vi "Mcp2210 Get Spi Status.vi"(8 "error in (no error)":errorcluster, 11 "handle":i32) -> (0 "error out":errorcluster, 2 "SPI Status":T1, 3 "handle out":i32)   [LabVIEW 2015, in "mcp2210.lvlib"]
doc: "If there is no device communication error, this command returns 0 (E_SUCCESS) and\nupdates the pointers with information about SPI transfer status. In case of error, the function\nreturns negative error code.\nParameters:\nInputs:\n- void *handle - The pointer to the USB device handle. Cannot be NULL.\nOutputs:\n- unsigned char *pspiExtReqStat - SPI Bus release external request status:\n- 0x01 ¨C No External Request for SPI Bus Release\n- 0x00 ¨C Pending External Request for SPI Bus Release\nCannot be NULL.\n- unsigned char *pspiOwner - SPI Bus current owner:\n- 0x00 - No owner\n- 0x01 - USB Bridge\n- 0x02 - External Master.\nCannot be NULL.\n- unsigned char *pspiTxferStat - SPI transfer status:\n- 0x00 - No SPI transfer in progress\n- 0x01 - SPI transfer is in progress\nCannot be NULL.\nReturns:\n- 0 for success: E_SUCCESS\n- negative error code: E_ERR_NULL, E_ERR_INVALID_HANDLE_VALUE\nE_ERR_HID_TIMEOUT, E_ERR_HID_RW_FILEIO, E_ERR_UNKOWN_ERROR\nE_ERR_CMD_ECHO, E_ERR_CMD_FAILED\n\nMCP2210_DLL_UM_API int __stdcall Mcp2210_GetSpiStatus(void *handle, unsigned char *pspiExtReqStat, unsigned char *pspiOwner, unsigned char *pspiTxferStat);"
uses:
  <userlib>/mcp2210/mcp2210.lvlib
  <userlib>/mcp2210/mcp2210_dll_um_x86.dll
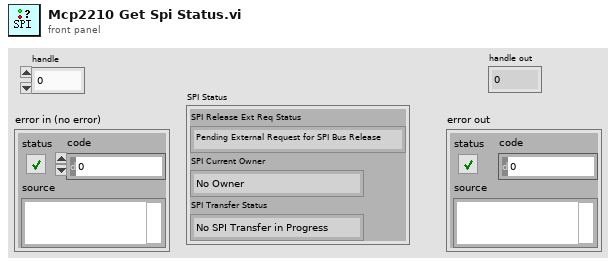
[diagram p1: front panel]
types:
  T1 = cluster{"SPI Release Ext Req Status":enum16{"Pending External Request for SPI Bus Release", "No External Request for SPI Bus Release"}, "SPI Current Owner":enum16{"No Owner", "USB Bridge", "External Master"}, "SPI Transfer Status":enum16{"No SPI Transfer in Progress", "SPI Transfer in Progress"}}
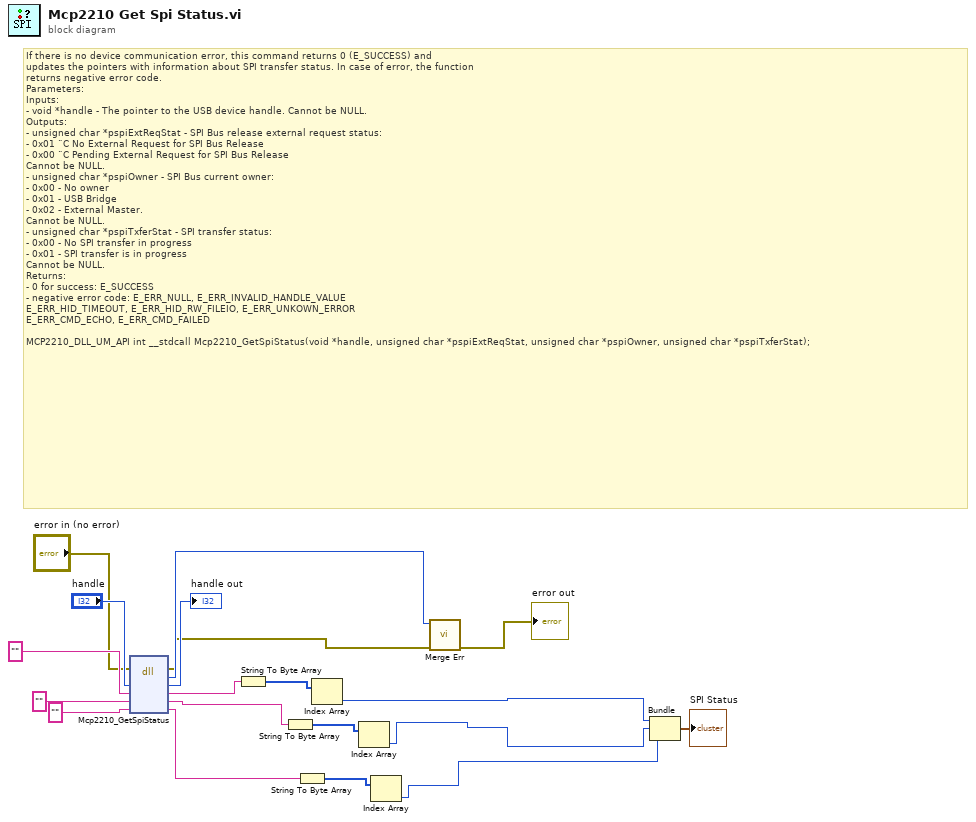
[diagram p0: block diagram]
diagram:
  # "If there is no device communication error, this command returns 0 (E_SUCCESS) and\nupdates the pointers with information about SPI transfer status. In case of error, the function\nreturns negative error code.\nParameters:\nInputs:\n- void *handle - The pointer to the USB device handle. Cannot be NULL.\nOutputs:\n- unsigned char *pspiExtReqStat - SPI Bus release external request status:\n- 0x01 ¨C No External Request for SPI Bus Release\n- 0x00 ¨C Pending External Request for SPI Bus Release\nCannot be NULL.\n- unsigned char *pspiOwner - SPI Bus current owner:\n- 0x00 - No owner\n- 0x01 - USB Bridge\n- 0x02 - External Master.\nCannot be NULL.\n- unsigned char *pspiTxferStat - SPI transfer status:\n- 0x00 - No SPI transfer in progress\n- 0x01 - SPI transfer is in progress\nCannot be NULL.\nReturns:\n- 0 for success: E_SUCCESS\n- negative error code: E_ERR_NULL, E_ERR_INVALID_HANDLE_VALUE\nE_ERR_HID_TIMEOUT, E_ERR_HID_RW_FILEIO, E_ERR_UNKOWN_ERROR\nE_ERR_CMD_ECHO, E_ERR_CMD_FAILED\n\nMCP2210_DLL_UM_API int __stdcall Mcp2210_GetSpiStatus(void *handle, unsigned char *pspiExtReqStat, unsigned char *pspiOwner, unsigned char *pspiTxferStat);"
  n1 = dll-call lib="D:/LabVIEW 2015/user.lib/mcp2210/mcp2210_dll_um_x86.*" fn="Mcp2210_GetSpiStatus"(error in="error in (no error)", "handle"="handle", "pspiExtReqStat"="", "pspiOwner"="", "pspiTxferStat"="") -> (error out=w13:errorcluster, "return type"=w14:i32, "handle"=→"handle out":i32, "pspiExtReqStat"=w10:string, "pspiOwner"=w7:string, "pspiTxferStat"=w5:string)  [unwired: 2 in, 1 out]
  n2 = String To Byte Array(string=w10) -> (unsigned byte array=w9:u8[])
  n3 = String To Byte Array(string=w7) -> (unsigned byte array=w8:u8[])
  n4 = String To Byte Array(string=w5) -> (unsigned byte array=w6:u8[])
  n5 = Index Array(array=w9) -> (element=w4:u8)  [unwired: 1 in]
  n6 = Index Array(array=w8) -> (element=w3:u8)  [unwired: 1 in]
  n7 = Index Array(array=w6) -> (element=w2:u8)  [unwired: 1 in]
  n8 = call <userlib>:"Merge Err.vi"("error in (no error)"=w13, "return type"=w14) -> ("error out"=→"error out":errorcluster)  [unwired: 9 in]
  n9 = Bundle(w4, w3, w2) -> (→"SPI Status":cluster{u8, u8, u8})  [unwired: 1 in]
